vi "Driving.vi"(11 "output cluster":T1) -> ()   [LabVIEW 2016]
uses:
  Joystick/ControlsToCommands.ctl
  References/Refnums.vi
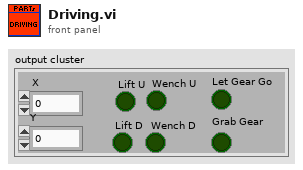
[diagram p1: front panel]
types:
  T1 = typedef "ControlsToCommands.ctl" = cluster{"X":dbl, "Y":dbl, "Lift U":bool, " Wench U":bool, " Wench D":bool, "Lift D":bool, "Let Gear Go":bool, "Grab Gear":bool}
  T2 = typedef "WPI_MotorControlDeviceRef.ctl" = cluster{"DeviceStatus":errorcluster, "Type":T3, "PWM":cluster{"PWM Channel":T4, "DeadBand":T5}, "CAN":cluster{"Device Number":u8, "SetOutput VI Ref":variant, "GetOutput VI Ref":variant, "Enable VI Ref":variant, "Disable VI Ref":variant, "Data":variant}, "Invert":bool}
  T3 = typedef "WPI_MotorControlType.ctl" = enum16{"PWM", "CAN"}
  T4 = typedef "FPGA_DIOPWMChannel.ctl" = enum8{"PWM 0", "PWM 1", "PWM 2", "PWM 3", "PWM 4", "PWM 5", "PWM 6", "PWM 7", "PWM 8", "PWM 9", "PWM MXP 0", "PWM MXP 1", "PWM MXP 2", "PWM MXP 3", "PWM MXP 4", "PWM MXP 5", "PWM MXP 6", "PWM MXP 7", "PWM MXP 8", "PWM MXP 9", "Invalid"}
  T5 = typedef "WPI_PWMDeadband.ctl" = cluster{"Name":string, "maxPositivePwm":i32, "minPositivePwm":i32, "centerPwm":i32, "maxNegativePwm":i32, "minNegativePwm":i32, "angularRange":u16}
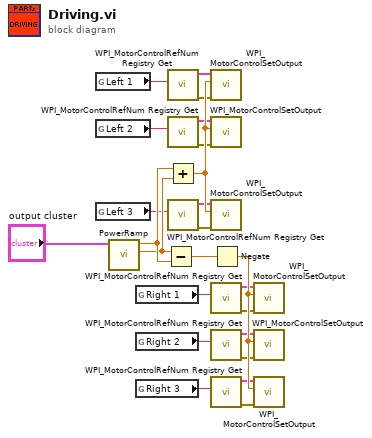
[diagram p0: block diagram]
diagram:
  n1 = global read "Refnums.vi" "Left 1"() -> (w18:string)
  n2 = global read "Refnums.vi" "Left 2"() -> (w17:string)
  n3 = global read "Refnums.vi" "Left 3"() -> (w12:string)
  n4 = call "PowerRamp.vi"("input cluster"="output cluster") -> ("Y"=w21:dbl, "X"=w24:dbl)  [unwired: 9 in]
  n5 = global read "Refnums.vi" "Right 1"() -> (w5:string)
  n6 = global read "Refnums.vi" "Right 2"() -> (w6:string)
  n7 = global read "Refnums.vi" "Right 3"() -> (w11:string)
  n8 = Subtract(x=w21, y=w24) -> (x-y=w1:dbl)
  n9 = call <vilib>:"WPI_MotorControlRefNum Registry Get.vi"("refnum name"=w18) -> ("error out"=w20:errorcluster, "MotorControlDevRef"=w19:T2)  [unwired: 9 in]
  n10 = call <vilib>:"WPI_MotorControlRefNum Registry Get.vi"("refnum name"=w17) -> ("error out"=w15:errorcluster, "MotorControlDevRef"=w16:T2)  [unwired: 9 in]
  n11 = Add(x=w24, y=w21) -> (x+y=w23:dbl)
  n12 = call <vilib>:"WPI_MotorControlRefNum Registry Get.vi"("refnum name"=w12) -> ("error out"=w14:errorcluster, "MotorControlDevRef"=w13:T2)  [unwired: 9 in]
  n13 = call <vilib>:"WPI_MotorControlSetOutput.vi"("error in (no error)"=w20, "Output"=w23, "MotorControlDevRef"=w19) -> ()  [unwired: 6 in, 3 out]
  n14 = call <vilib>:"WPI_MotorControlSetOutput.vi"("error in (no error)"=w15, "Output"=w23, "MotorControlDevRef"=w16) -> ()  [unwired: 6 in, 3 out]
  n15 = call <vilib>:"WPI_MotorControlSetOutput.vi"("error in (no error)"=w14, "Output"=w23, "MotorControlDevRef"=w13) -> ()  [unwired: 6 in, 3 out]
  n16 = call <vilib>:"WPI_MotorControlRefNum Registry Get.vi"("refnum name"=w5) -> ("error out"=w3:errorcluster, "MotorControlDevRef"=w4:T2)  [unwired: 9 in]
  n17 = call <vilib>:"WPI_MotorControlRefNum Registry Get.vi"("refnum name"=w6) -> ("error out"=w8:errorcluster, "MotorControlDevRef"=w7:T2)  [unwired: 9 in]
  n18 = call <vilib>:"WPI_MotorControlRefNum Registry Get.vi"("refnum name"=w11) -> ("error out"=w9:errorcluster, "MotorControlDevRef"=w10:T2)  [unwired: 9 in]
  n19 = Negate(x=w1) -> (-x=w22:dbl)
  n20 = call <vilib>:"WPI_MotorControlSetOutput.vi"("error in (no error)"=w3, "Output"=w22, "MotorControlDevRef"=w4) -> ()  [unwired: 6 in, 3 out]
  n21 = call <vilib>:"WPI_MotorControlSetOutput.vi"("error in (no error)"=w8, "Output"=w22, "MotorControlDevRef"=w7) -> ()  [unwired: 6 in, 3 out]
  n22 = call <vilib>:"WPI_MotorControlSetOutput.vi"("error in (no error)"=w9, "Output"=w22, "MotorControlDevRef"=w10) -> ()  [unwired: 6 in, 3 out]
